vi "fpga_Signal_rise_detection.vi"(1 "Signal IN":bool) -> (0 "Signal change LOW->HIGH?":bool)   [LabVIEW 2011]
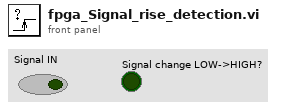
[diagram p1: front panel]
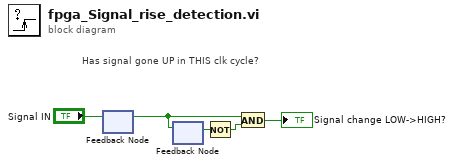
[diagram p0: block diagram]
diagram:
  # "Has signal gone UP in THIS clk cycle?"
  n1 = feedback-in #1("Signal IN") -> ()
  n2 = feedback #1() -> (w1:bool)  [unwired: 1 in]
  n3 = feedback #2() -> (w5:bool)  [unwired: 1 in]
  n4 = feedback-in #2(w1) -> ()
  n5 = Not(x=w5) -> (.not. x?=w3:bool)
  n6 = And(x=w1, y=w3) -> (x .and. y?=→"Signal change LOW->HIGH?":bool)
